vi "PlanetMaker_SubVI.vi"(5 "Color":u32(colorbox), 7 "Detail":sgl=1.0, 8 "error in (no error)":errorcluster, 9 "Name":string, 10 "Translation":cluster{"X":sgl, "Y":sgl, "Z":sgl}, 11 "Radius":sgl=1.0) -> (0 "error out":errorcluster, 3 "Rotated Scene Object":refnum<vi>)   [LabVIEW 2015]
uses:
  <vilib>/picture/3D Picture Control/NI_3D Picture Control.lvlib
  <vilib>/picture/3D Picture Control/Object/Create Object (drawable).vi
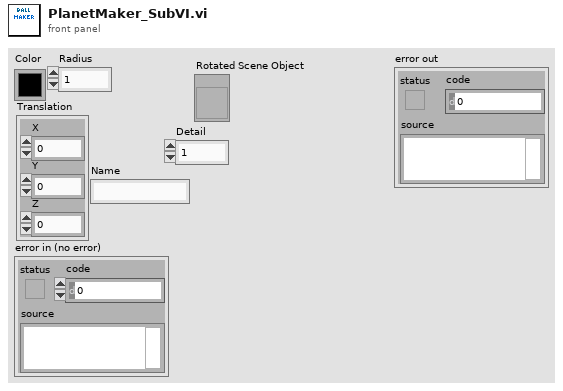
[diagram p1: front panel]
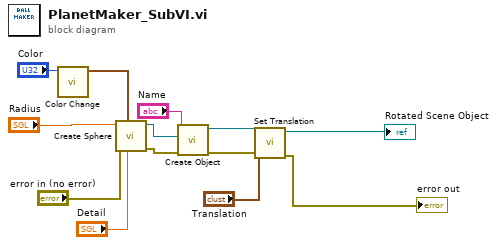
[diagram p0: block diagram]
diagram:
  n1 = call <vilib>:"Color Change.vi"("Color"="Color") -> ("RGBA"=w13:cluster{"R":sgl, "G":sgl, "B":sgl, "A":sgl})  [unwired: 10 in]
  n2 = call <vilib>:"Create Sphere.vi"("Detail"="Detail", "Color"=w13, "error in (no error)"="error in (no error)", "Radius"="Radius") -> ("error out"=w9:errorcluster, "New Sphere Refnum"=w10:refnum<vi>)  [unwired: 6 in]
  n3 = call-poly <vilib>:"Create Object.vi"("error in (no error)"=w9, "Geometry"=w10, "Name"="Name") -> ("error out"=w7:errorcluster, "Scene:New Object"=w8:refnum<vi>)  [unwired: 7 in]
  n4 = call <vilib>:"Set Translation.vi"("error in (no error)"=w7, "Translation"="Translation", "Scene Object"=w8) -> ("error out"=→"error out":errorcluster, "Translated Object"=→"Rotated Scene Object":refnum<vi>)  [unwired: 7 in]
